vi "Close.vi"(8 "error in (no error)":errorcluster, 11 "MelsecTCP in":refnum<class "InovanceSerial.lvclass">) -> (0 "error out":errorcluster, 3 "MelsecTCP out":refnum<class "InovanceSerial.lvclass">)   [LabVIEW 2020, in "HslCommunication.lvlib" / "InovanceSerial.lvclass"]
uses:
  InovanceSerial.lvclass
  Read reference.vi
  D:/Git/Labview-Libraries/Libraries/HslCommunication/_Dependenciecs/HslCommunication.dll
  _Dependenciecs/HslCommunication.dll
  InovanceSerial.lvclass/InovanceSerial.ctl
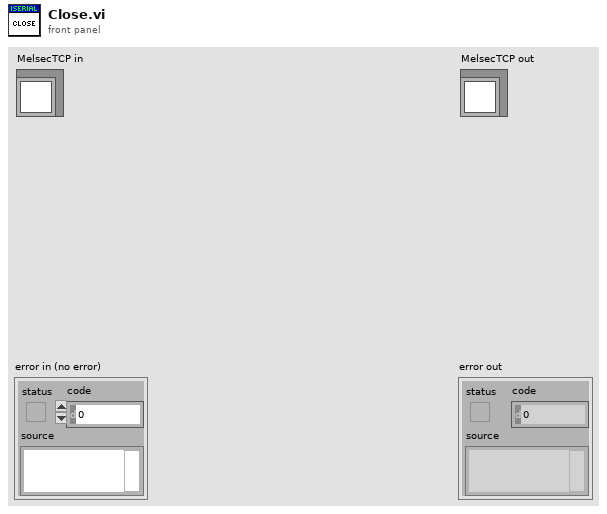
[diagram p1: front panel]
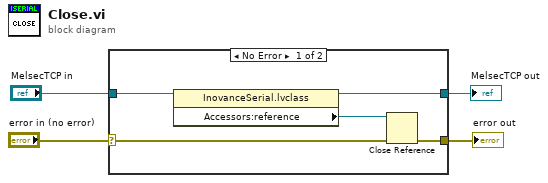
[diagram p0: block diagram]
diagram:
  n1 = case shown="No Error" "error in (no error)" {
    selector: "error in (no error)" -> [w8 w11]
    tunnel: "MelsecTCP in" -> [w9 w10]
    tunnel: [w7 w10] -> w2
    tunnel: [w6 w11] -> w1
    frame No Error {
      n2 = property class="InovanceSerial.lvclass"(reference=w9) -> (reference out=w7:refnum<class "InovanceSerial.lvclass">, "Accessors:reference"=w5:refnum<k24>)  [unwired: 1 in, 1 out]
      n3 = Close Reference(reference=w5, error in (no error)=w8) -> (error out=w6:errorcluster)
    }
    frame Error {
    }
  }
  "error out" <- w1
  "MelsecTCP out" <- w2
